vi "refresh table model.vi"(6 "Filter":string, 7 "engine configuration":refnum<class "engine configuration.lvclass">, 8 "error in":errorcluster, 9 "avail tags":refnum<vi>, 10 "chan table":refnum<vi>, 11 "TDMS datalogger configuration":refnum<class "TDMS datalogger configuration.lvclass">) -> (0 "error out":errorcluster, 3 "TDMS datalogger configuration out":refnum<class "TDMS datalogger configuration.lvclass">, 5 "engine configuration out":refnum<class "engine configuration.lvclass">)   [LabVIEW 2015, in "TDMS datalogger editor node.lvclass"]
uses:
  TDMS datalogger editor node.lvclass
  module/configuration/TDMS datalogger configuration.lvclass
  <vilib>/NI/Module Execution Interface/Engine Configuration/engine configuration.lvclass
  <vilib>/NI/Configuration Framework/serializable configuration/NISE_CEF_serializable configuration.lvclass/NISE_CEF_serializable configuration.ctl
  module/configuration/TDMS datalogger configuration.lvclass/TDMS datalogger configuration.ctl
  <vilib>/NI/Tag Bus/tag/tag descriptor.lvclass/tag descriptor.ctl
  <vilib>/NI/Module Execution Interface/Engine Configuration/engine configuration.lvclass/engine configuration.ctl
  <vilib>/NI/Tag Bus/tag/write tag name.vi
  <vilib>/NI/Tag Bus/tag/read tag name.vi
  <vilib>/NI/Tag Bus/tag/read data type.vi
  <vilib>/NI/Configuration Framework/serializable configuration/Read UID.vi
  module/configuration/Read channels.vi
  <vilib>/Utility/LVClass/Get LV Class Name.vi
  <vilib>/NI/Configuration Framework/error generator/NISE_error generator.vi
  Table Items.vi
  <vilib>/NI/Tag Bus Module Framework/channel/TBM channel.lvclass
  <vilib>/NI/Tag Bus/tag/tag descriptor.lvclass
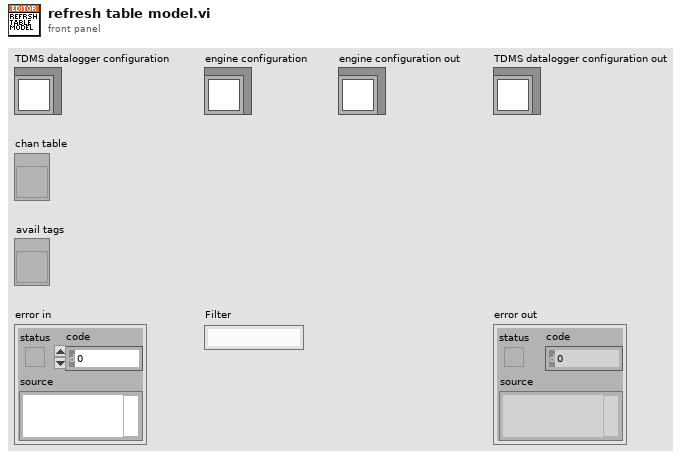
[diagram p1: front panel]
types:
  T1 = typedef "tag bus.lvlib/tag descriptor.lvclass/Data Type.ctl" = enum16{"Double", "Single", "I64", "I32", "I16", "I8", "U64", "U32", "U16", "U8", "Boolean", "String", "Array of Double", "Array of Single", "Array of I64", "Array of I32", "Array of I16", "Array of I8", "Array of U64", "Array of U32", "Array of U16", "Array of U8", "Array of Boolean", "Array of String"}
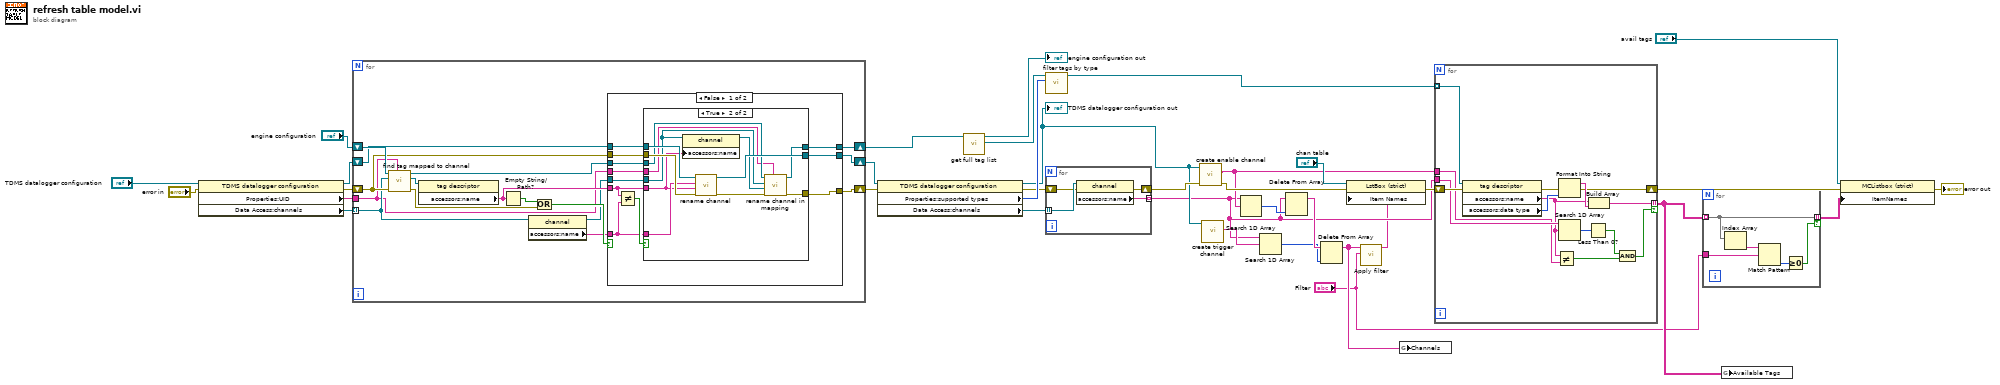
[diagram p0: block diagram]
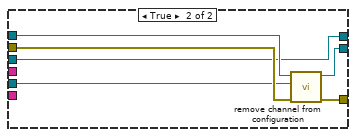
[diagram p3: hidden frame]
diagram:
  n1 = property class="TDMS datalogger configuration"(reference="TDMS datalogger configuration", error in="error in") -> (reference out=w30:refnum<class "TDMS datalogger configuration.lvclass">, error out=w32:errorcluster, "Properties:UID"=w26:string, "Data Access:channels"=w33:refnum<class "TBM channel.lvclass">[])
  n2 = for {
    tunnel: w33 -> [w43] mode=indexing
    shift-right: [w38] -> w16
    shift-left: "engine configuration" -> [w51]
    shift-right: [w48] -> w29
    shift-left: w30 -> [w46]
    tunnel: w26 -> [w37]
    shift-right: [w47] -> w28
    shift-left: w32 -> [w44]
    n3 = call <vilib>:"find tag mapped to channel.vi"("owner"=w37, "error in"=w44, "channel"=w43, "engine configuration in"=w51) -> ("error out"=w42:errorcluster, "tag"=w50:refnum<class "tag descriptor.lvclass">, "engine configuration out"=w39:refnum<class "engine configuration.lvclass">)  [unwired: 5 in]
    n4 = property class="tag descriptor"(reference=w50) -> ("accessors:name"=w40:string)  [unwired: 1 in, 2 out]
    n5 = Empty String/Path?(string/path=w40) -> (empty?=w49:bool)
    n6 = property class="channel"(reference=w43) -> (reference out=w36:refnum<class "TBM channel.lvclass">, "accessors:name"=w41:string)  [unwired: 1 in, 1 out]
    n7 = Or(x=w49, y=w42) -> (x .or. y?=w45:bool)
    n8 = case shown="False" w45 {
      tunnel: [w59 w83] -> w48
      tunnel: [w62 w82] -> w47
      tunnel: w44 -> [w61 w81]
      tunnel: w46 -> [w60 w80]
      tunnel: w36 -> [w52 w79]
      tunnel: w41 -> [w57 _]
      tunnel: w40 -> [w56 _]
      tunnel: w39 -> [w55 w78]
      tunnel: [w54 w78] -> w38
      tunnel: w37 -> [w53 _]
      frame False {
        n9 = Not Equal?(x=w56, y=w57) -> (x != y?=w58:bool)
        n10 = case shown="True" w58 {
          tunnel: [w65 w70] -> w62
          tunnel: w61 -> [w65 w76]
          tunnel: w60 -> [w64 w77]
          tunnel: [w64 w75] -> w59
          tunnel: w57 -> [_ w74]
          tunnel: w56 -> [_ w67]
          tunnel: w55 -> [w63 w73]
          tunnel: [w63 w72] -> w54
          tunnel: w53 -> [_ w69]
          tunnel: w52 -> [_ w68]
          frame False {
          }
          frame True {
            n11 = property class="channel"(reference=w68, "accessors:name"=w67) -> (reference out=w66:refnum<class "TBM channel.lvclass">)  [unwired: 1 in, 1 out]
            n12 = call "rename channel.vi"("error in"=w76, "new name"=w67, "old name"=w74, "TDMS datalogger configuration in"=w77) -> ("error out"=w71:errorcluster, "TDMS datalogger configuration out"=w75:refnum<class "TDMS datalogger configuration.lvclass">)  [unwired: 6 in]
            n13 = call <vilib>:"rename channel in mapping.vi"("owner ID"=w69, "error in"=w71, "new channel"=w66, "old channel"=w68, "engine configuration in"=w73) -> ("error out"=w70:errorcluster, "engine configuration out"=w72:refnum<class "engine configuration.lvclass">)  [unwired: 5 in]
          }
        }
      }
      frame True {
        n14 = call "remove channel from configuration.vi"("error in"=w81, "TBM channel in"=w79, "TDMS datalogger configuration in"=w80) -> ("error out"=w82:errorcluster, "TDMS datalogger configuration out"=w83:refnum<class "TDMS datalogger configuration.lvclass">)  [unwired: 7 in]
      }
    }
  }
  n15 = property class="TDMS datalogger configuration"(reference=w29, error in=w28) -> (reference out=w10:refnum<class "TDMS datalogger configuration.lvclass">, error out=w24:errorcluster, "Properties:supported types"=w27:T1[], "Data Access:channels"=w25:refnum<class "TBM channel.lvclass">[])
  "TDMS datalogger configuration out" <- w10
  n16 = call <vilib>:"get full tag list.vi"("engine configuration in"=w16) -> ("tag list"=w14:refnum<class "tag descriptor.lvclass">[], "engine configuration out"=→"engine configuration out":refnum<class "engine configuration.lvclass">)  [unwired: 9 in]
  n17 = call <vilib>:"filter tags by type.vi"("allowable types"=w27, "tags in"=w14) -> ("filtered tags"=w22:refnum<class "tag descriptor.lvclass">[])  [unwired: 9 in]
  n18 = for {
    tunnel: w25 -> [w87] mode=indexing
    shift-right: [w86] -> w13
    shift-left: w24 -> [w85]
    tunnel: [w84] -> w7 mode=indexing
    n19 = property class="channel"(reference=w87, error in=w85) -> (error out=w86:errorcluster, "accessors:name"=w84:string)  [unwired: 1 out]
  }
  n20 = call "create enable channel.vi"("error in"=w13, "TDMS datalogger configuration"=w10) -> ("error out"=w12:errorcluster, "enable channel name"=w11:string)  [unwired: 7 in, 1 out]
  n21 = call "create trigger channel.vi"("TDMS datalogger configuration"=w10) -> ("trigger channel name"=w8:string)  [unwired: 8 in, 2 out]
  n22 = Search 1D Array(1D array=w7, element=w11) -> (index of element=w23:i32)  [unwired: 1 in]
  n23 = Search 1D Array(1D array=w7, element=w8) -> (index of element=w6:i32)  [unwired: 1 in]
  n24 = Delete From Array(array=w7, index=w23) -> (array with subset deleted=w9:string[])  [unwired: 1 in, 1 out]
  n25 = Delete From Array(array=w9, index=w6) -> (array with subset deleted=w4:string[])  [unwired: 1 in, 1 out]
  n26 = call "Apply filter.vi"("Filter"="Filter", "Item names"=w4) -> ("Filtered Item Names"=w5:string[])  [unwired: 9 in]
  n27 = property class="LstBox (strict)"(reference="chan table", error in=w12, "Item Names"=w5) -> (error out=w21:errorcluster)  [unwired: 1 out]
  n28 = global write "Table Items.vi" "Channels"(w4) -> ()
  n29 = for {
    tunnel: w22 -> [w99] mode=indexing
    shift-right: [w96] -> w20
    shift-left: w21 -> [w98]
    tunnel: [w95] -> w3 mode=indexing if=w91
    tunnel: w7 -> [w94]
    tunnel: w11 -> [w90]
    n30 = property class="tag descriptor"(reference=w99, error in=w98) -> (error out=w97:errorcluster, "accessors:name"=w88:string, "accessors:data type"=w100:T1)  [unwired: 1 out]
    n31 = Not Equal?(x=w88, y=w90) -> (x != y?=w89:bool)
    n32 = Format Into String(error in=w97, w100) -> (resulting string=w101:string, error out=w96:errorcluster)  [unwired: 2 in]
    n33 = Search 1D Array(1D array=w94, element=w88) -> (index of element=w93:i32)  [unwired: 1 in]
    n34 = Less Than 0?(x=w93) -> (x < 0?=w92:bool)
    n35 = Build Array(w88, w101) -> (w95:string[])
    n36 = Compound Arithmetic op=AND(w92, w89) -> (w91:bool)
  }
  n37 = for {
    tunnel: w3 -> [w103] mode=indexing
    tunnel: "Filter" -> [w104]
    tunnel: [w103] -> w2 mode=indexing if=w102
    n38 = Index Array(array=w103) -> (element=w105:string)  [unwired: 1 in]
    n39 = Match Pattern(string=w105, regular expression=w104) -> (offset past match=w106:i32)  [unwired: 1 in, 3 out]
    n40 = Greater Or Equal To 0?(x=w106) -> (x >= 0?=w102:bool)
  }
  n41 = global write "Table Items.vi" "Available Tags"(w3) -> ()
  n42 = property class="MCListbox (strict)"(reference="avail tags", error in=w20, "ItemNames"=w2) -> (error out=→"error out":errorcluster)  [unwired: 1 out]
